vi "立方根（牛顿迭代法）.vi"() -> ()   [LabVIEW 2012]
doc: "功能：\n\n利用牛顿迭代法求一个数的立方根\n\n\ncsxcs_366创建"
panel:
  out "cube root(x)":dbl
  in  "a":dbl
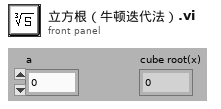
[diagram p1: front panel]
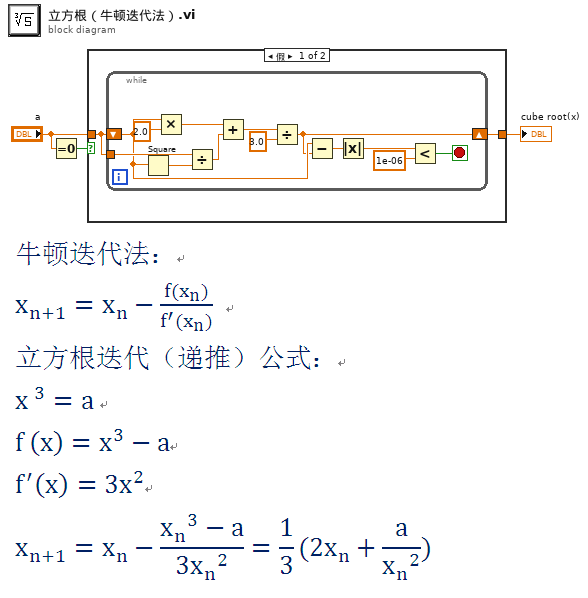
[diagram p0: block diagram]
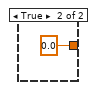
[diagram p2: hidden frame]
diagram:
  n1 = Equal To 0?(x="a") -> (x = 0?=w2:bool)
  n2 = case shown="假" w2 {
    tunnel: "a" -> [w5 _]
    tunnel: [w4 0.0 ("x")] -> w1
    frame False {
      n3 = while {
        tunnel: w5 -> [w13]
        shift-right: [w6] -> w4
        shift-left: w5 -> [w12]
        stop <- w15 stop-if-true
        n4 = Square(x=w12) -> (x^2=w14:dbl)
        n5 = Multiply(x=w12, y=2.0) -> (x*y=w9:dbl)
        n6 = Divide(x=w13, y=w14) -> (x/y=w10:dbl)
        n7 = Add(x=w9, y=w10) -> (x+y=w8:dbl)
        n8 = Divide(x=w8, y=3.0) -> (x/y=w6:dbl)
        n9 = Subtract(x=w12, y=w6) -> (x-y=w18:dbl)
        n10 = Absolute Value(x=w18) -> (abs(x)=w17:dbl)
        n11 = Less?(x=w17, y=1e-06) -> (x < y?=w15:bool)
      }
    }
    frame True {
    }
  }
  "cube root(x)" <- w1
